vi "Write5WirexVDTParameters.vi"(8 "error in (no error)":errorcluster, 9 "UserValues":dbl[](array[numeric]), 10 "5 Wire xVDT Parameters in":T1[](array[typedef]), 11 "FPGA Session":u32) -> (0 "error out":errorcluster, 2 "5 Wire xVDT Parameters out":T1[](array[typedef]), 3 "FPGA Session Out":u32)   [LabVIEW 2011, in "Sensor Simulation Custom Device.lvlib"]
uses:
  Sensor Simulation Custom Device.lvlib
  TypeDefs/5 Wire xVDT Parameters.ctl
  <userlib>/_FPGA Interface Advanced Tools/FPGA Interface Wrapper/NiFPGA Write - I32.vi
  <vilib>/Utility/error.llb/Error Cluster From Error Code.vi
  <userlib>/_FPGA Interface Advanced Tools/FPGA Interface Wrapper/FPGA Interface Wrapper.lvlib
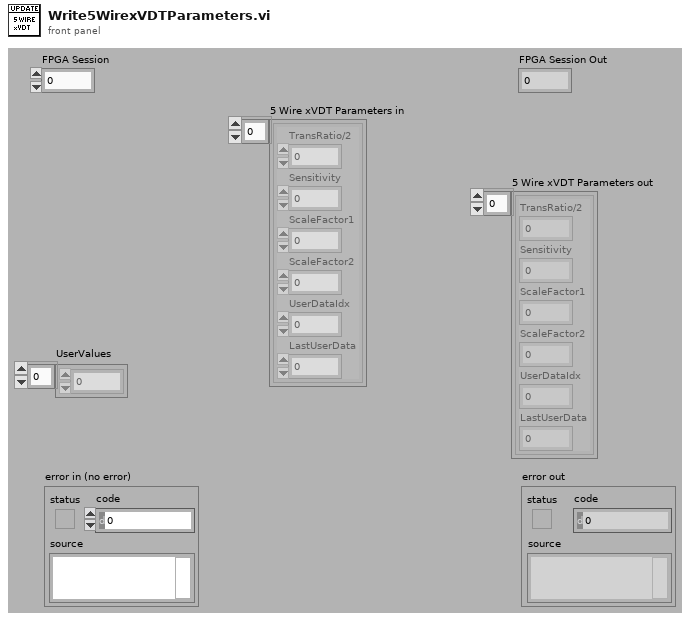
[diagram p1: front panel]
types:
  T1 = typedef "Sensor Simulation Custom Device.lvlib/5 Wire xVDT Parameters.ctl" = cluster{"TransRatio/2":dbl, "Sensitivity":dbl, "ScaleFactor1":u32, "ScaleFactor2":u32, "UserDataIdx":i32, "LastUserData":dbl}
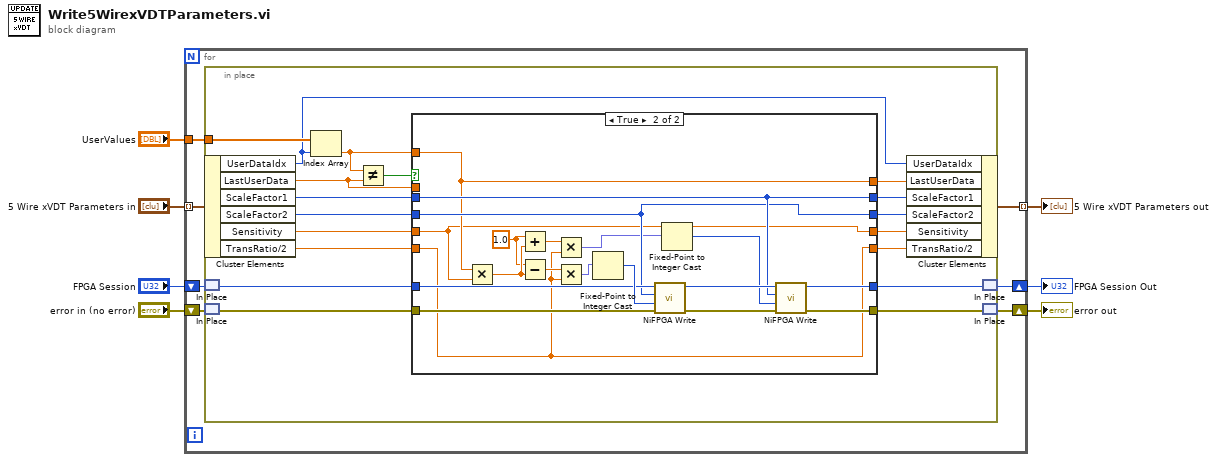
[diagram p0: block diagram]
diagram:
  n1 = for {
    shift-right: [w11] -> w6
    shift-left: "error in (no error)" -> [w12]
    shift-right: [w10] -> w5
    shift-left: "FPGA Session" -> [w13]
    tunnel: "5 Wire xVDT Parameters in" -> [w9] mode=indexing
    tunnel: "UserValues" -> [w14]
    tunnel: [w8] -> w1 mode=indexing
    n2 = in-place {
      in-place-border: w14 -> [w32]
      n3 = in-place-cluster #1(w9) -> ("UserDataIdx"=w23:i32, "LastUserData"=w24:dbl, "ScaleFactor1"=w22:u32, "ScaleFactor2"=w21:u32, "Sensitivity"=w20:dbl, "TransRatio/2"=w19:dbl)
      n4 = in-place-match #2(w13) -> (w31:u32)
      n5 = in-place-match #3(w12) -> (w30:errorcluster)
      n6 = Index Array(array=w32, index=w23) -> (element=w26:dbl)
      n7 = Not Equal?(x=w26, y=w24) -> (x != y?=w27:bool)
      n8 = case shown="True" w27 {
        tunnel: w31 -> [w38 w54]
        tunnel: w30 -> [w37 w53]
        tunnel: [w37 w52] -> w29
        tunnel: [w38 w51] -> w28
        tunnel: w19 -> [w36 w40]
        tunnel: w20 -> [w35 w47]
        tunnel: w21 -> [w34 w49]
        tunnel: w22 -> [w33 w50]
        tunnel: w26 -> [_ w48]
        tunnel: [w39 w48] -> w25
        tunnel: w24 -> [w39 _]
        tunnel: [w36 w40] -> w18
        tunnel: [w35 w47] -> w17
        tunnel: [w34 w49] -> w16
        tunnel: [w33 w50] -> w15
        frame False {
        }
        frame True {
          w41 = 1.0 ("x")
          n9 = Multiply(x=w48, y=w47) -> (x*y=w45:dbl)
          n10 = Add(x=w41, y=w45) -> (x+y=w43:dbl)
          n11 = Subtract(x=w41, y=w45) -> (x-y=w46:dbl)
          n12 = Multiply(x=w43, y=w40) -> (x*y=w42:fxp<+/-,19,5>)
          n13 = Multiply(x=w46, y=w40) -> (x*y=w44:fxp<+/-,19,5>)
          n14 = Fixed-Point to Integer Cast(1:w44) -> (0:w57:i32)
          n15 = call-poly <userlib>:"NiFPGA Write.vi"("error in (no error)"=w53, "Value"=w57, "Control"=w49, "Session"=w54) -> ("error out"=w58:errorcluster, "Session Out"=w56:u32)  [unwired: 6 in]
          n16 = Fixed-Point to Integer Cast(1:w42) -> (0:w55:i32)
          n17 = call-poly <userlib>:"NiFPGA Write.vi"("error in (no error)"=w58, "Value"=w55, "Control"=w50, "Session"=w56) -> ("error out"=w52:errorcluster, "Session Out"=w51:u32)  [unwired: 6 in]
        }
      }
      n18 = in-place-cluster #1("UserDataIdx"=w23, "LastUserData"=w25, "ScaleFactor1"=w15, "ScaleFactor2"=w16, "Sensitivity"=w17, "TransRatio/2"=w18) -> (w8:T1)
      n19 = in-place-match #2(w28) -> (w10:u32)
      n20 = in-place-match #3(w29) -> (w11:errorcluster)
    }
  }
  "error out" <- w6
  "FPGA Session Out" <- w5
  "5 Wire xVDT Parameters out" <- w1
